vi "TestRobotic.vi"() -> ()   [LabVIEW 2017]
uses:
  <vilib>/robotics/Controls/Simulator Display/Simulator Display.xctl
  <vilib>/robotics/Simulator/Engine/ctl/Step Mode.ctl
  <vilib>/Analysis/_algsub.llb/Real Vector Norm.vi
  <vilib>/robotics/Kinematics/Analytical/SCARA/NI_Robotics_SCARA Serial Arm Class.lvclass
  C:/Program Files (x86)/National Instruments/LabVIEW 2017/vi.lib/robotics/Kinematics/Robot/NI_Robotics_Serial Robot Arm.lvclass
  <vilib>/robotics/Kinematics/Analytical/SCARA/Initialize SCARA Serial Arm.vi
  <vilib>/robotics/Kinematics/Robot/Forward Kinematics (Point).vi
  <vilib>/robotics/Kinematics/Generate Joint Trajectory (Int).vi
  <vilib>/robotics/Kinematics/NI_Kinematics.lvlib
  <vilib>/robotics/Kinematics/Analytical/NI_Robotics_AnalyticKinematics.lvlib
  <vilib>/Analysis/NI_AALPro.lvlib
  <vilib>/robotics/Simulator/NI_Robotics_Simulator.lvlib
  C:/Program Files (x86)/National Instruments/LabVIEW 2017/vi.lib/robotics/Kinematics/Analytical/Generic/NI_Robotics_Analytical Serial Arm Class.lvclass
panel:
  in  "Simulator Display":refnum<vi>(xcontrol)
  out "appended path":path
  in  "Manifest Filename":string="SCARA Arm.xml"
  out "X":dbl
  out "Y":dbl
  out "max(x,y)":dbl
  out "x":dbl
  out "y":dbl
  out "Boolean":bool
  out "x+1":dbl
  out "joint position trajectory":dbl[][](array[numeric])
  out "subarray":dbl[](array[numeric])
  out "joint position trajectory 3":dbl[][](array[numeric])
  out "Arm Joints 2":dbl[](array[numeric])
  out "x-y":dbl[](array[numeric])
  out "NaN/Path/Refnum?":bool
  out "joint positions":dbl[][](array[numeric])
  in  "End Effector Posture 3":dbl[](array[slide])=[1.0, -3.6739403974420595e-17, 0.6000000000000001, 0.0] scale=-1.0..1.0
  out "Truoc":dbl[](array[numeric])
  out "HienTai":dbl[](array[numeric])
  in  "End Effector Posture":T1 {"theta" scale=-3.14..3.14; "Z" scale=0.25..0.75}
  out "appended array":dbl[](array[numeric])
  out "Arm Joints":dbl[](array[slide])=[0.5235980365896387, -1.5691963261122304, 1.0455982895225908, 0.0] scale=-3.0..3.0
  out "translation vector":dbl[](array[numeric])
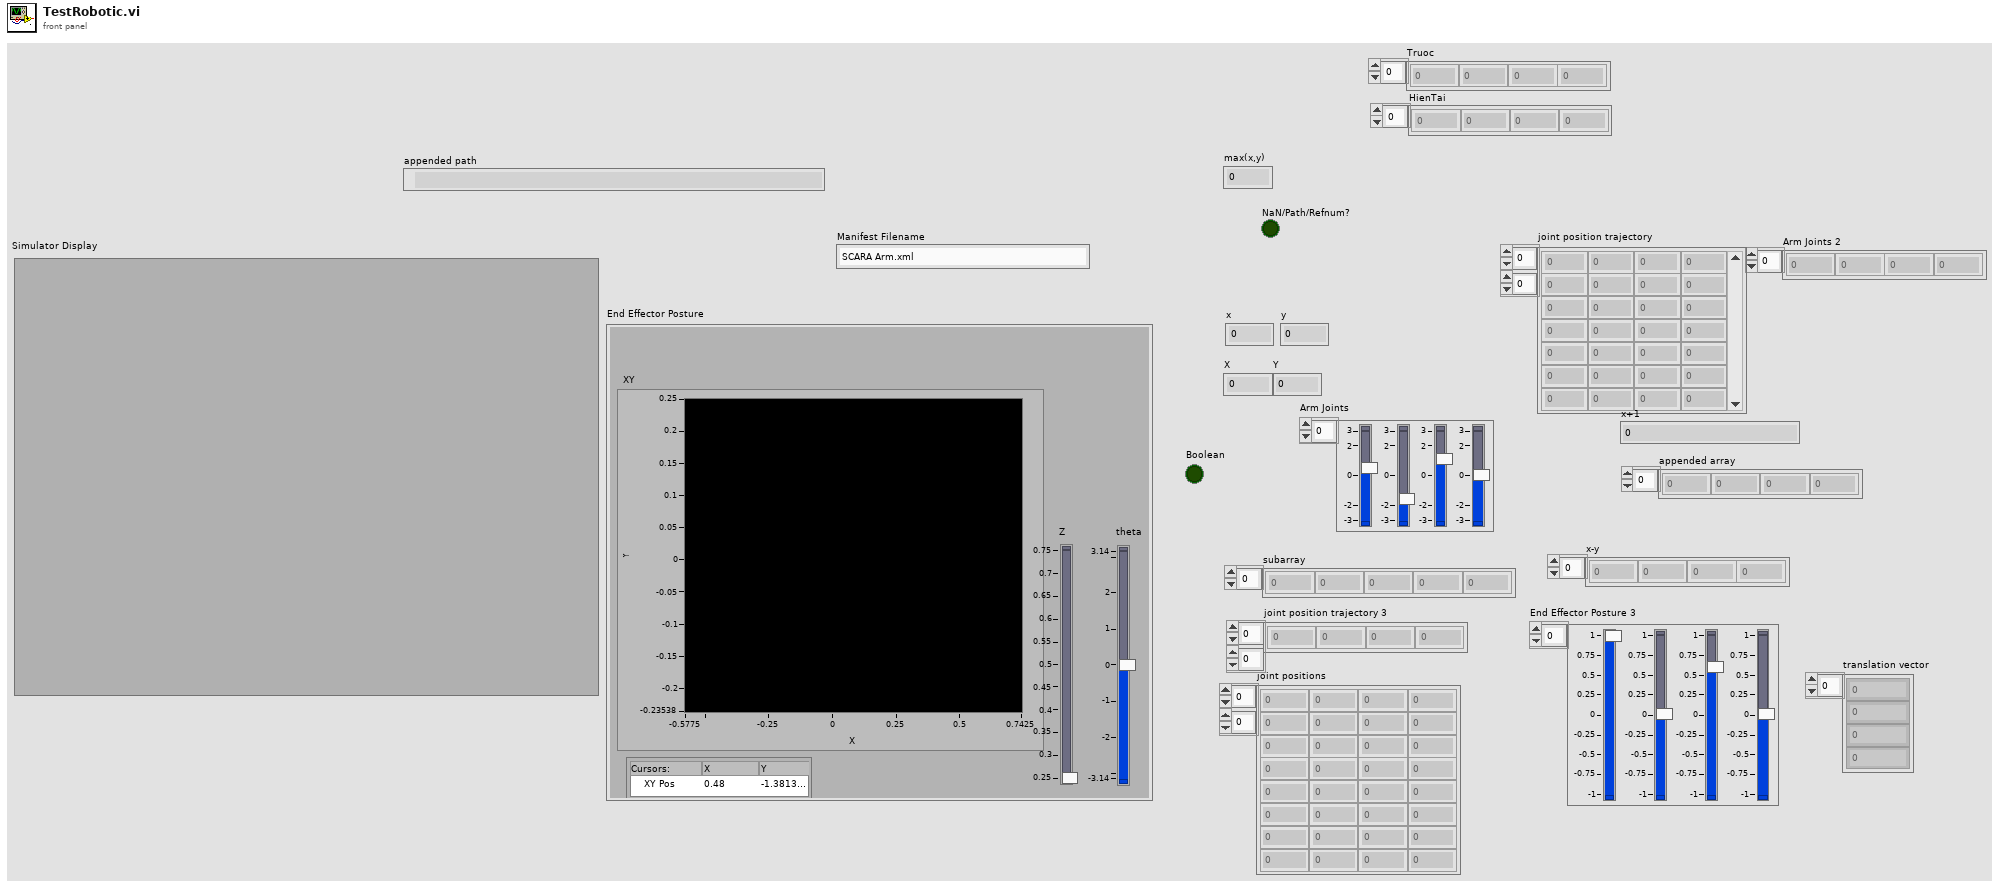
[diagram p1: front panel]
types:
  T1 = cluster{"XY":cluster{"X":dbl, "Y":dbl}[], "Z":dbl, "theta":dbl}
  T2 = typedef "NI_Robotics_Simulator.lvlib/Step Mode.ctl" = u16
  T3 = typedef "NI_Matrix.lvlib/RealMatrix.ctl" = dbl[][]
  T4 = typedef "LVPointDoubleTypeDef.ctl" = cluster{"Cursor X":dbl, "Cursor Y":dbl}
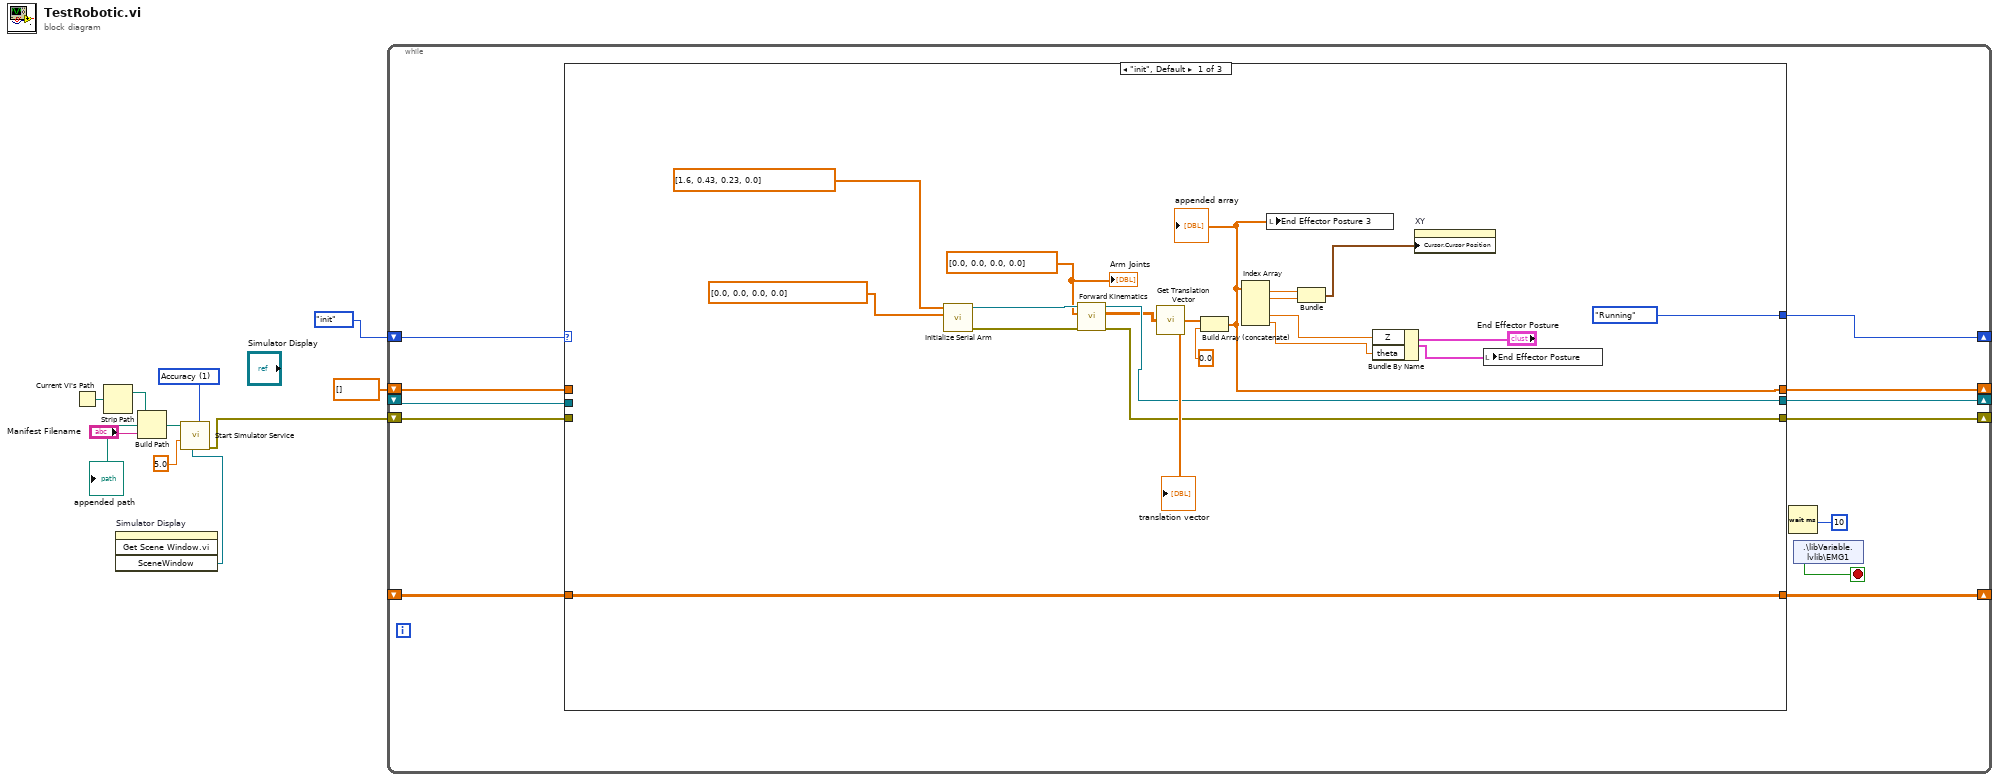
[diagram p0: block diagram]
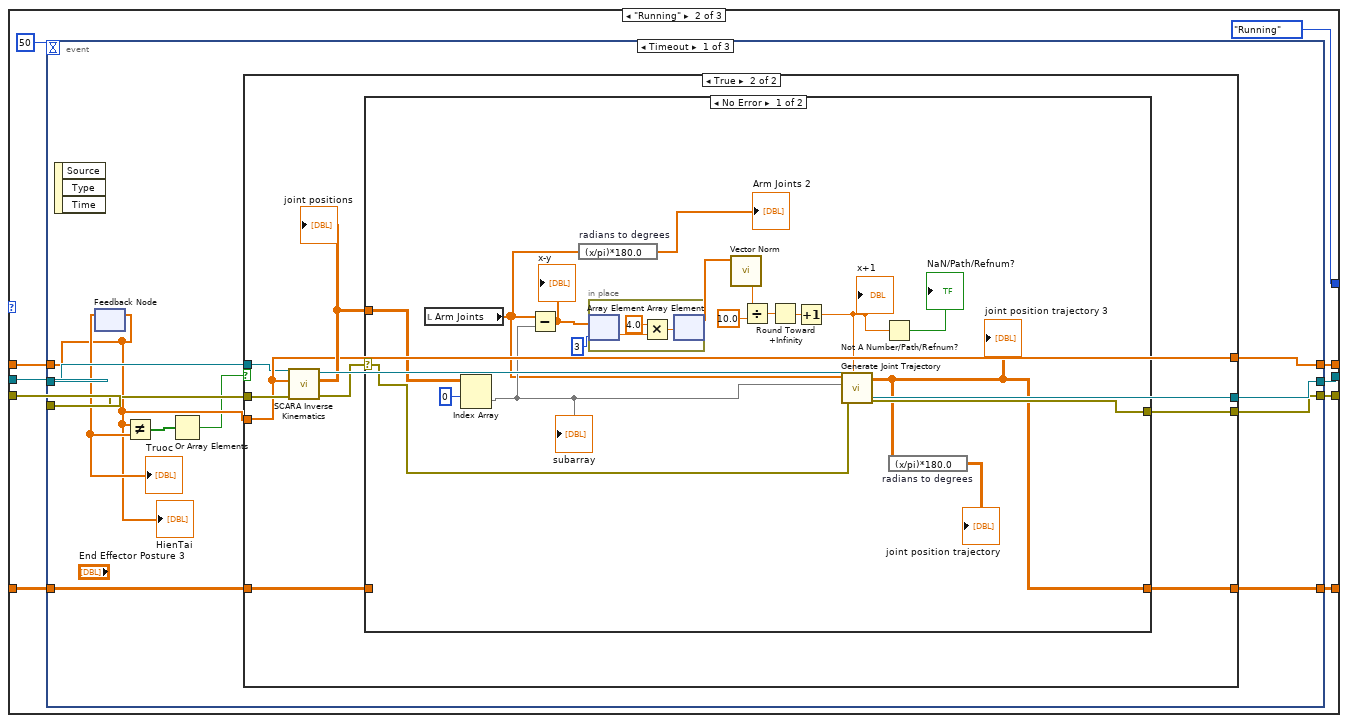
[diagram p2: hidden frame]
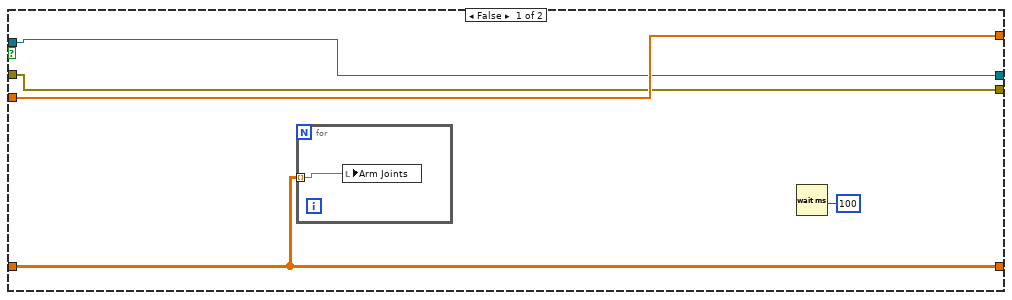
[diagram p3: hidden frame]
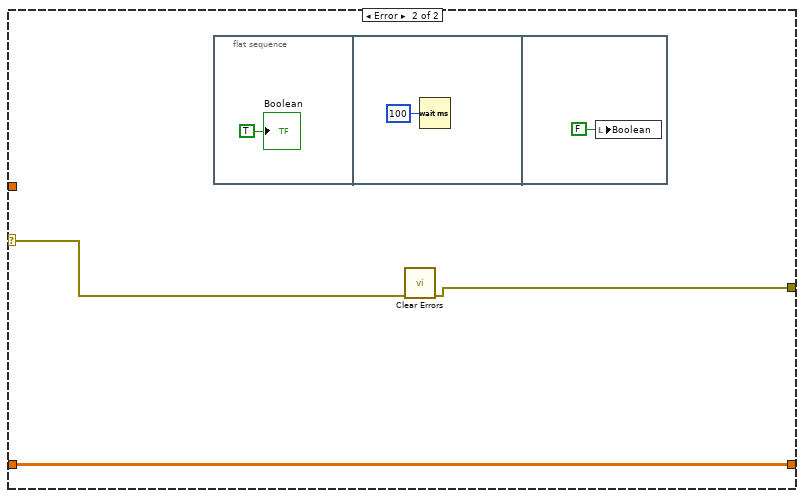
[diagram p4: hidden frame]
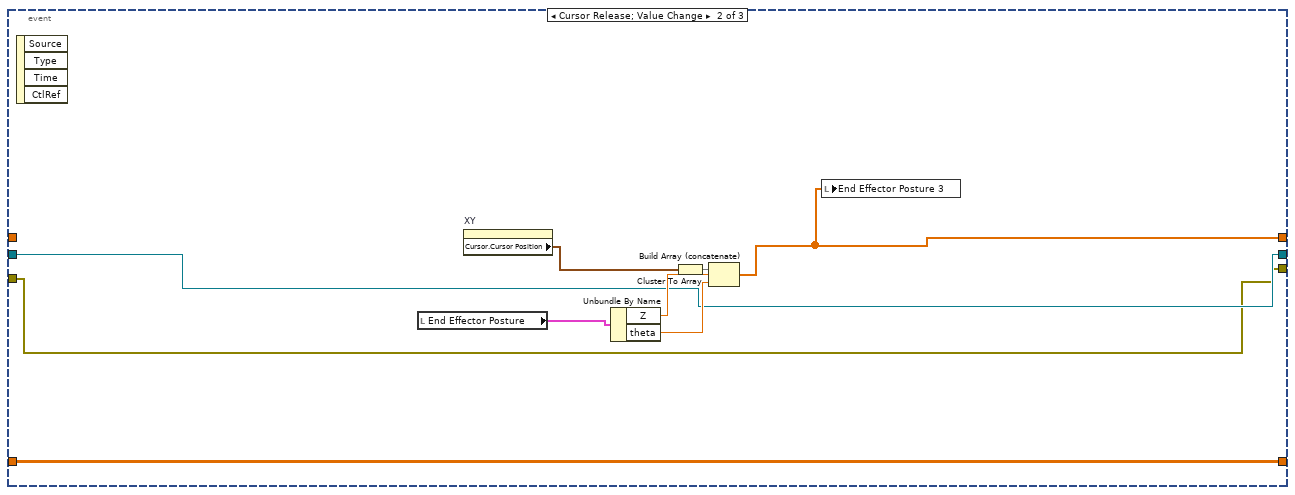
[diagram p5: hidden frame]
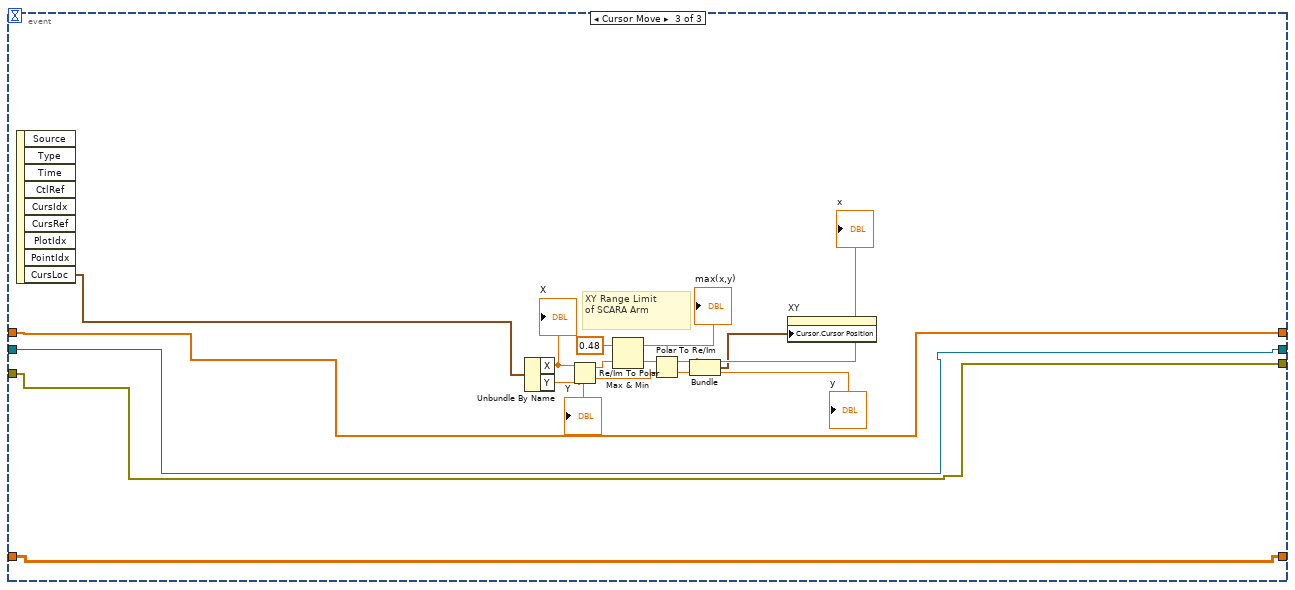
[diagram p6: hidden frame]
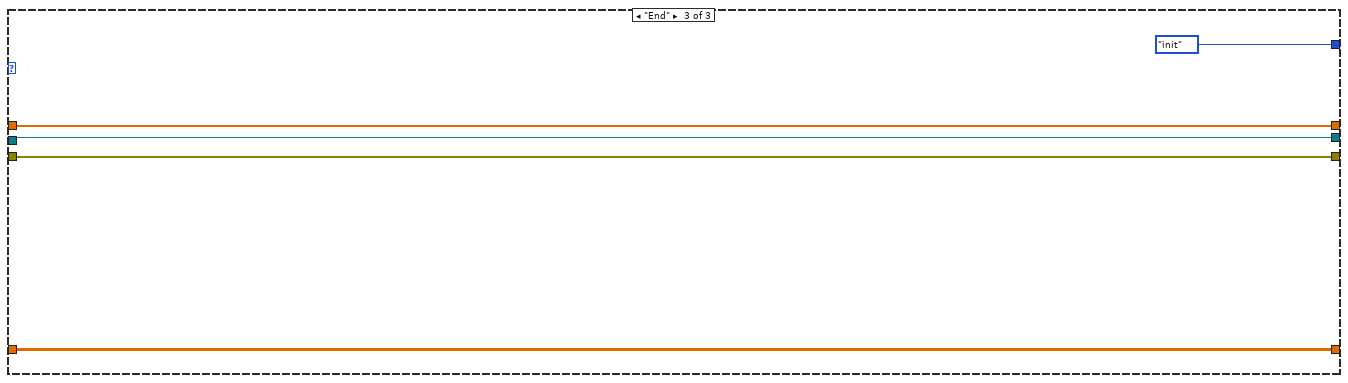
[diagram p7: hidden frame]
diagram:
  w3 = T2 1 items=["Performance", "Accuracy"] ("step mode")
  n1 = Current VI's Path() -> (path=w7:path)
  n2 = Strip Path(path=w7) -> (stripped path=w6:path)  [unwired: 1 out]
  n3 = invoke on="Simulator Display" class="Simulator Display (strict)" method="Get Scene Window.vi"() -> ("SceneWindow"=w1:refnum<vi>)  [unwired: 4 in, 3 out]
  n4 = Build Path(base path=w6, name or relative path="Manifest Filename") -> (appended path=w5:path)
  "appended path" <- w5
  n5 = call <vilib>:"Start Simulator Service.vi"("step mode"=w3, "3D picture refnum"=w1, "step size (ms)"=5.0 ("stepsize(ms)"), "manifest file"=w5) -> ("error out"=w2:errorcluster)  [unwired: 7 in]
  n6 = while {
    shift-right: [w19] -> _
    shift-left: enum16{"init", "Running", "End"}."init" -> [w20]
    shift-right: [w18] -> _
    shift-left: _ -> [w16]
    shift-right: [w17] -> _
    shift-left: w2 -> [w15]
    shift-right: [w13] -> _
    shift-left: dbl[] [] -> [w14]
    shift-right: [w12] -> _
    shift-left: _ -> [w11]
    stop <- w21 stop-if-true
    n7 = case shown="\"init\", Default" w20 {
      tunnel: [enum16{"init", "Running", "End"}."Running" enum16{"init", "Running", "End"}."Running" enum16{"init", "Running", "End"}."init"] -> w19
      tunnel: [w28 w49 w133] -> w18
      tunnel: [w26 w47 w132] -> w17
      tunnel: w16 -> [_ w51 w133]
      tunnel: w15 -> [_ w50 w132]
      tunnel: w14 -> [_ w46 w131]
      tunnel: [w24 w45 w131] -> w13
      tunnel: [w34 w44 w130] -> w12
      tunnel: w11 -> [w34 w43 w130]
      frame "init", Default {
        w23 = dbl[] [0.0, 0.0, 0.0, 0.0] ("Offsets")
        n8 = call-poly <vilib>:"Initialize Serial Arm.vi"("offsets"=dbl[] [0.0, 0.0, 0.0, 0.0] ("Offsets"), "lengths"=dbl[] [1.6, 0.43, 0.23, 0.0] ("Lengths")) -> ("error out"=w29:errorcluster, "SCARA serial arm out"=w30:refnum<class "NI_Robotics_SCARA Serial Arm Class.lvclass">)  [unwired: 8 in]
        n9 = call-poly <vilib>:"Forward Kinematics.vi"("error in (no error)"=w29, "joint positions"=w23, "serial arm in"=w30) -> ("error out"=w26:errorcluster, "end effector transform"=w27:T3, "serial arm out"=w28:refnum<class "NI_Robotics_SCARA Serial Arm Class.lvclass">)  [unwired: 6 in]
        n10 = call <vilib>:"Get Translation Vector.vi"("transform"=w27) -> ("translation vector"=w41:dbl[])
        "translation vector" <- w41
        n11 = Build Array (concatenate)(w41, 0.0) -> (w24:dbl[])
        "appended array" <- w24
        n12 = Index Array(array=w24) -> (element #1=w39:dbl, element #2=w38:dbl, element #3=w37:dbl, element #4=w36:dbl)  [unwired: 4 in]
        n13 = local write "End Effector Posture 3"(w24) -> ()
        n14 = Bundle("Numeric"=w39, "Numeric"=w38) -> (w25:cluster{"Numeric":dbl, "Numeric":dbl})  [unwired: 1 in]
        n15 = Bundle By Name(cluster="End Effector Posture", "Z"=w37, "theta"=w36) -> (w33:T1)
        n16 = property on="XY" class="XYGraph (strict)"("Cursor.Cursor Position"=w25) -> ()  [unwired: 2 in, 2 out]
        n17 = local write "End Effector Posture"(w33) -> ()
        "Arm Joints" <- w23
      }
      frame "Running" {
        n18 = event shown="[0] Timeout" {
          selector: _ -> [_ _ _]
          dyn-events: _ -> [_ _ _]
          timeout: 50 -> [_ _ _]
          tunnel: w51 -> [w59 w108 w119]
          tunnel: w50 -> [w63 w107 w118]
          tunnel: [w62 w108 w119] -> w49
          tunnel: [w61 w107 w118] -> w47
          tunnel: w46 -> [w54 _ w120]
          tunnel: [w60 w106 w120] -> w45
          tunnel: [w57 w109 w117] -> w44
          tunnel: w43 -> [w56 w109 w117]
          event Timeout {
            n19 = event-data() -> ()  [unwired: 1 in, 3 out]
            n20 = feedback-in #1(w54) -> ()
            n21 = feedback #1() -> (w55:dbl[])  [unwired: 1 in]
            "Truoc" <- w55
            n22 = Not Equal?(x=w54, y=w55) -> (x != y?=w58:bool[])
            n23 = Or Array Elements(Boolean array=w58) -> (logical OR=w53:bool)
            n24 = case shown="True" w53 {
              tunnel: w63 -> [w66 w78]
              tunnel: [w67 w77] -> w62
              tunnel: [w66 w76] -> w61
              tunnel: [w68 w74] -> w60
              tunnel: w54 -> [w68 w74]
              tunnel: w59 -> [w67 w73]
              tunnel: [w65 w72] -> w57
              tunnel: w56 -> [w65 w71]
              frame False {
                n25 = for {
                  tunnel: w65 -> [w69] mode=indexing
                  n26 = local write "Arm Joints"(w69) -> ()
                }
                n27 = Wait (ms)(milliseconds to wait=u32 100) -> ()  [unwired: 1 out]
              }
              frame True {
                n28 = call <vilib>:"SCARA Inverse Kinematics.vi"("error in (no error)"=w78, "end effector position"=w74, "SCARA serial arm in"=w73) -> ("error out"=w70:errorcluster, "joint positions"=w75:dbl[][], "SCARA serial arm out"=w77:refnum<class "NI_Robotics_SCARA Serial Arm Class.lvclass">)  [unwired: 6 in]
                "joint positions" <- w75
                n29 = case shown="No Error" w70 {
                  selector: w70 -> [w85 w101]
                  tunnel: [w91 w102] -> w76
                  tunnel: w75 -> [w86 _]
                  tunnel: [w84 w100] -> w72
                  tunnel: w71 -> [_ w100]
                  frame No Error {
                    n30 = local read "Arm Joints"() -> (w82:dbl[])
                    n31 = Index Array(array=w86, index (row)=0) -> (element=w90:dbl[])  [unwired: 1 in]
                    "subarray" <- w90
                    n32 = Subtract(x=w82, y=w90) -> (x-y=w89:dbl[])
                    "x-y" <- w89
                    n33 = expression code="(x/pi)*180.0" "radians to degrees"(w82) -> (→"Arm Joints 2":dbl[])
                    n34 = in-place {
                      n35 = in-place-array #2(w89, 3) -> (w99:dbl)
                      n36 = Multiply(x=4.0, y=w99) -> (x*y=w97:dbl)
                      n37 = in-place-array #2(w97) -> (w87:dbl[])  [unwired: 1 out]
                    }
                    n38 = call-poly <vilib>:"Vector Norm.vi"("Input Vector"=w87) -> ("norm"=w95:dbl)  [unwired: 9 in, 1 out]
                    n39 = Divide(x=w95, y=10.0) -> (x/y=w93:dbl)
                    n40 = Round Toward +Infinity(x=w93) -> (ceil(x): smallest int >= x=w92:dbl)
                    n41 = Increment(x=w92) -> (x+1=w80:dbl)
                    "x+1" <- w80
                    n42 = call-poly <vilib>:"Generate Joint Trajectory.vi"("intermediate points"=w80, "error in (no error)"=w85, "end joint positions"=w90, "start joint positions"=w82) -> ("error out"=w91:errorcluster, "joint position trajectory"=w84:dbl[][])  [unwired: 4 in, 2 out]
                    "joint position trajectory 3" <- w84
                    n43 = Not A Number/Path/Refnum?(number/path/refnum=w80) -> (NaN/Path/Refnum?=→"NaN/Path/Refnum?":bool)
                    n44 = expression code="(x/pi)*180.0" "radians to degrees"(w84) -> (→"joint position trajectory":dbl[][])
                  }
                  frame Error {
                    n45 = flat-sequence {
                      frame #0 {
                        "Boolean" <- TRUE ("Boolean")
                      }
                      frame #1 {
                        n46 = Wait (ms)(milliseconds to wait=u32 100) -> ()  [unwired: 1 out]
                      }
                      frame #2 {
                        n47 = local write "Boolean"(FALSE ("Boolean")) -> ()
                      }
                    }
                    n48 = call <vilib>:"Clear Errors.vi"("error in (no error)"=w101) -> ("error out"=w102:errorcluster)  [unwired: 5 in, 1 out]
                  }
                }
              }
            }
            "HienTai" <- w54
          }
          event "End Effector Posture.XY": Cursor Release; "End Effector Posture.Z", "End Effector Posture.theta": Value Change {
            n49 = event-data() -> ()  [unwired: 1 in, 4 out]
            n50 = local read "End Effector Posture"() -> (w111:T1)
            n51 = property on="XY" class="XYGraph (strict)"() -> ("Cursor.Cursor Position"=w110:T4)  [unwired: 2 in, 2 out]
            n52 = Unbundle By Name(w111) -> ("Z"=w113:dbl, "theta"=w112:dbl)
            n53 = Cluster To Array(cluster=w110) -> (array=w114:dbl[])
            n54 = Build Array (concatenate)(w114, w113, w112) -> (w106:dbl[])
            n55 = local write "End Effector Posture 3"(w106) -> ()
          }
          event "End Effector Posture.XY": Cursor Move {
            # "XY Range Limit \nof SCARA Arm"
            n56 = event-data() -> ("CursLoc"=w121:cluster{"X":dbl, "Y":dbl})  [unwired: 1 in, 8 out]
            n57 = Unbundle By Name(w121) -> ("X"=w123:dbl, "Y"=w122:dbl)
            "X" <- w123
            "Y" <- w122
            n58 = Re/Im To Polar(2:w122, 3:w123) -> (0:w127:dbl, 1:w129:dbl)
            n59 = Max & Min(x=0.48, y=w129) -> (max(x,y)=→"max(x,y)":dbl, min(x,y)=w126:dbl)
            n60 = Polar To Re/Im(2:w127, 3:w126) -> (0:w124:dbl, 1:w125:dbl)
            "x" <- w125
            "y" <- w124
            n61 = Bundle(w125, w124) -> (w116:cluster{dbl, dbl})  [unwired: 1 in]
            n62 = property on="XY" class="XYGraph (strict)"("Cursor.Cursor Position"=w116) -> ()  [unwired: 2 in, 2 out]
          }
        }
      }
      frame "End" {
      }
    }
    n63 = Wait (ms)(milliseconds to wait=u32 10) -> ()  [unwired: 1 out]
    n64 = shared-variable ".\\libVariable.lvlib\\EMG1"() -> (w21:bool)  [unwired: 1 in, 1 out]
  }
